vi "rs3 get device info.vi"(8 "error in (no error)":errorcluster, 10 "RS Camera info":u16(ring) items=["    RS2_CAMERA_INFO_NAME                           , /**< Friendly name */", "    RS2_CAMERA_INFO_SERIAL_NUMBER                  , /**< Device serial number */", "    RS2_CAMERA_INFO_FIRMWARE_VERSION               , /**< Primary firmware version */", "    RS2_CAMERA_INFO_PHYSICAL_PORT                       , /**< Unique identifier of the port the device is connected to (platform specific) */", "    RS2_CAMERA_INFO_DEBUG_OP_CODE                  , /**< If device supports firmware logging, this is the command to send to get logs from firmware */", "    RS2_CAMERA_INFO_ADVANCED_MODE                  , /**< True iff the device is in advanced mode */", "    RS2_CAMERA_INFO_PRODUCT_ID                     , /**< Product ID as reported in the USB descriptor */", "    RS2_CAMERA_INFO_CAMERA_LOCKED                  , /**< True iff EEPROM is locked */", "    RS2_CAMERA_INFO_COUNT                            /**< Number of enumeration values. Not a valid input: intended to be used in for-loops. */"], 11 "device in":u64) -> (0 "error out":errorcluster, 1 "error":u64, 2 "info":string, 3 "device out":u64)   [LabVIEW 2017, in "libRealSense3.lvlib"]
doc: "Get the properties of a specific DEVICE. \n\nINPUT: \nDev in Device handle\nRS Camera info Drop-down menu of the information being requested\n\nOUTPUT:\nInfo String of info (for example, the Camera name, or serial number)\nError Error=0 is no error"
uses:
  libRealSense3.lvlib
  realsense2.dll
panel:
  # "RS3 Get Device Info"
  # "(C) 2017 Intel Corp.,  AGJ"
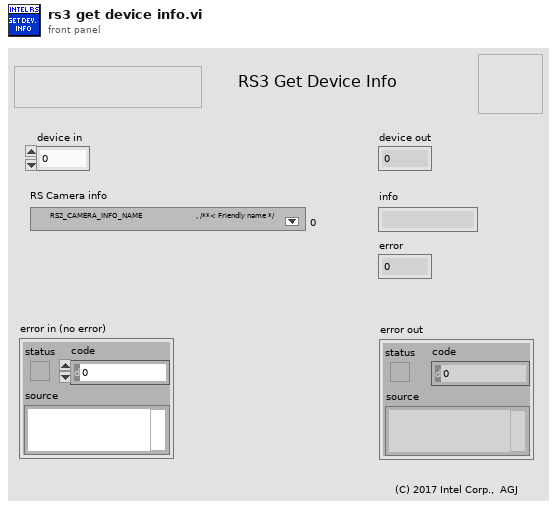
[diagram p1: front panel]
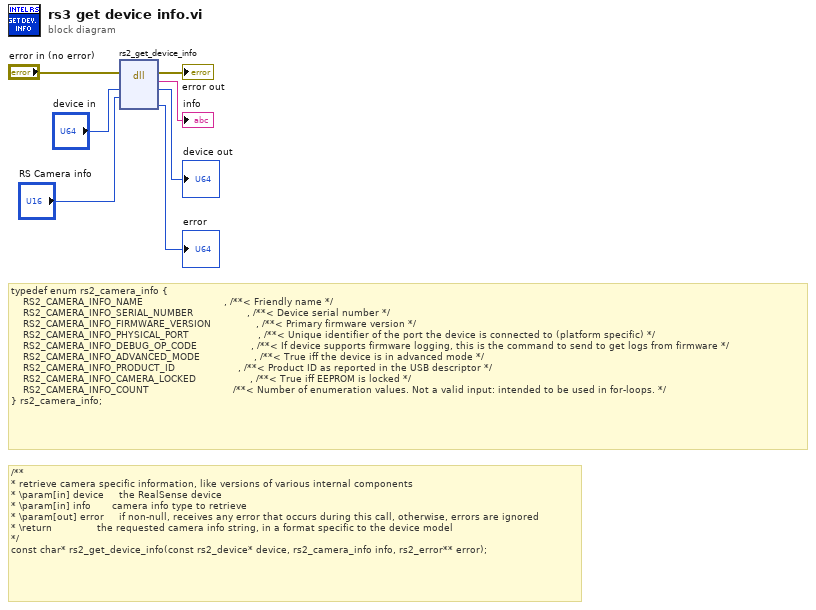
[diagram p0: block diagram]
diagram:
  # "typedef enum rs2_camera_info {\n    RS2_CAMERA_INFO_NAME                           , /**< Friendly name */\n    RS2_CAMERA_INFO_SERIAL_NUMBER                  , /**< Device serial number */\n    RS2_CAMERA_INFO_FIRMWARE_VERSION               , /**< Primary firmware version */\n    RS2_CAMERA_INFO_PHYSICAL_PORT                       , /**< Unique identifier of the port the device is connected to (platform specific) */\n    RS2_CAMERA_INFO_DEBUG_OP_CODE                  , /**< If device supports firmware logging, this is the command to send to get logs from firmware */\n    RS2_CAMERA_INFO_ADVANCED_MODE                  , /**< True iff the device is in advanced mode */\n    RS2_CAMERA_INFO_PRODUCT_ID                     , /**< Product ID as reported in the USB descriptor */\n    RS2_CAMERA_INFO_CAMERA_LOCKED                  , /**< True iff EEPROM is locked */\n    RS2_CAMERA_INFO_COUNT                            /**< Number of enumeration values. Not a valid input: intended to be used in for-loops. */\n} rs2_camera_info;"
  # "/**\n* retrieve camera specific information, like versions of various internal components\n* \\param[in] device     the RealSense device\n* \\param[in] info       camera info type to retrieve\n* \\param[out] error     if non-null, receives any error that occurs during this call, otherwise, errors are ignored\n* \\return               the requested camera info string, in a format specific to the device model\n*/\nconst char* rs2_get_device_info(const rs2_device* device, rs2_camera_info info, rs2_error** error);"
  n1 = dll-call lib="C:/Users/smartek/Desktop/labview/realsense2.dll" fn="rs2_get_device_info"(error in="error in (no error)", "device"="device in", "info"="RS Camera info") -> (error out=→"error out":errorcluster, "Device name"=→"info":string, "device"=→"device out":u64, "error"=→"error":u64)  [unwired: 4 in, 1 out]
